vi "Split String To I32 Spreadsheet Array_Uti.vi"(2 "StringIn":string) -> (7 "Array":dbl[](array[numeric]), 9 "Default":dbl)   [LabVIEW 2012]
doc: "字符串格式为1,2,3;4，将\";\"前的字符以\",\"为分隔拆分为一个数组输出，将\";\"后的字符作为默认值输出。"
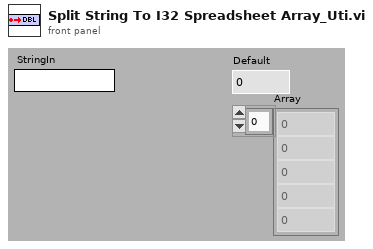
[diagram p1: front panel]
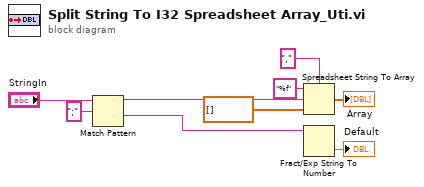
[diagram p0: block diagram]
diagram:
  n1 = Match Pattern(string="StringIn", regular expression=";") -> (before substring=w7:string, after substring=w6:string)  [unwired: 3 out]
  n2 = Spreadsheet String To Array(delimiter (Tab)=",", format string="%f", spreadsheet string=w7, array type (2D Dbl)=dbl[] [] ("Volts1/Div")) -> (array=→"Array":dbl[])
  n3 = Fract/Exp String To Number(string=w6) -> (number=→"Default":dbl)  [unwired: 3 in, 1 out]
